vi "Temperature Monitor.vi"() -> ()   [LabVIEW 2014]
doc: "本VI每间隔1秒采集温度值。本VI也计算最近5次温度测量值的平均值，并通过波形图表显示原始数据和实时平均值。本VI将原始数据保存至文本文件中。"
panel:
  in  "停止按钮":bool
  out "温度历史":cluster{dbl, "Temperature Value":dbl}(graph)
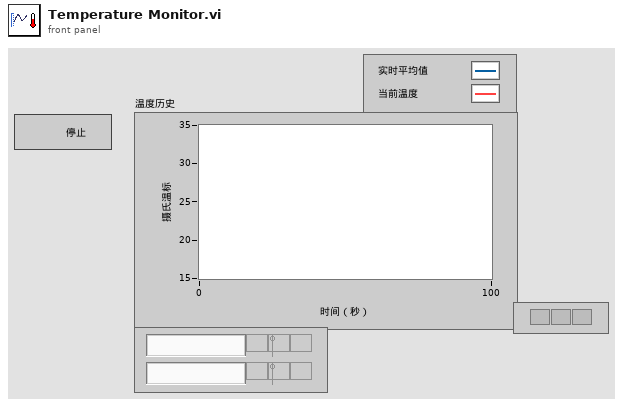
[diagram p1: front panel]
types:
  T1 = enum16{"open", "replace", "create", "open or create", "replace or create", "replace or create with confirmation"}
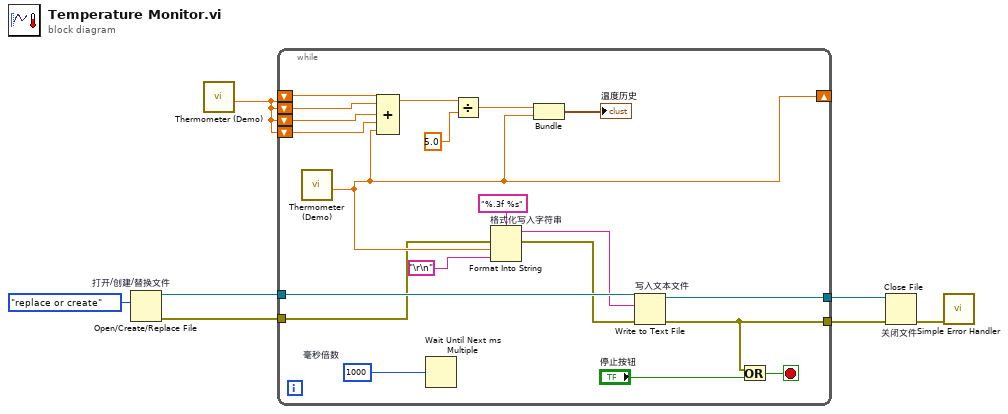
[diagram p0: block diagram]
diagram:
  n1 = Open/Create/Replace File "打开/创建/替换文件"(operation (0:open)=T1."replace or create" ("操作(0:open)")) -> (refnum out=w2:refnum<file>, error out=w4:errorcluster)  [unwired: 1 in, 5 out]
  n2 = call "Thermometer (Demo).vi"() -> ("温度值"=w7:dbl)  [unwired: 11 in]
  n3 = while {
    shift-right: [w13] -> _
    shift-left: w7 -> [w26]
    shift-left: w7 -> [w25]
    shift-left: w7 -> [w22]
    shift-left: w7 -> [w21]
    tunnel: w4 -> [w11]
    tunnel: [w16] -> w3
    tunnel: w2 -> [w18]
    tunnel: [w17] -> w1
    stop <- w14 stop-if-true
    w27 = u32 1000  # 毫秒倍数
    n4 = call "Thermometer (Demo).vi"() -> ("温度值"=w13:dbl)  [unwired: 11 in]
    n5 = Compound Arithmetic op=ADD(w26, w25, w22, w21, w13) -> (w24:dbl)
    n6 = Wait Until Next ms Multiple(millisecond multiple=w27) -> ()  [unwired: 1 out]
    n7 = Divide(x=w24, y=5.0) -> (x/y=w20:dbl)
    n8 = Format Into String "格式化写入字符串"(format string="%.3f %s" ("格式字符串"), error in=w11, w13, "\r\n" ("行结束常量")) -> (resulting string=w12:string, error out=w10:errorcluster)  [unwired: 1 in]
    n9 = Bundle(w20, "温度值"=w13) -> (→"温度历史":cluster{dbl, "温度值":dbl})  [unwired: 1 in]
    n10 = Write to Text File "写入文本文件"(file (use dialog)=w18, text=w12, error in=w10) -> (refnum out=w17:refnum<file>, error out=w16:errorcluster)  [unwired: 2 out]
    n11 = Or(x=w16, y="停止按钮") -> (x .or. y?=w14:bool)
  }
  n12 = Close File "关闭文件"(refnum=w1, error in=w3) -> (error out=w5:errorcluster)  [unwired: 1 out]
  n13 = call <vilib>:"Simple Error Handler.vi"("error in (no error)"=w5) -> ()  [unwired: 1 in, 8 out]
